vi "GetDefaultParams.vi"(8 "error in (no error)":errorcluster, 10 "Path":path, 11 "PmuTestFunctions.lvclass":refnum<class "PmuTestFunctions.lvclass">) -> (0 "error out":errorcluster, 3 "PmuTestFunctions.lvclass":refnum<class "PmuTestFunctions.lvclass">)   [LabVIEW 2014, in "Functions.lvlib" / "PmuTestFunctions.lvclass"]
uses:
  PmuTestFunctions.lvclass
  Typedefs/PmuTestParams.ctl
  FunctionBaseClass/FunctionBase.lvclass/FunctionBase.ctl
  PmuTestFunctions.lvclass/PmuTestFunctions.ctl
  FunctionBaseClass/Accessors/Read FunctionIniFilePath.vi
  Accessors/Write PmuTestParams.vi
  Accessors/Write T0.vi
  ArbitraryFunction/ArbitraryFunction.lvclass
  <vilib>/Utility/config.llb/NI_LVConfig.lvlib
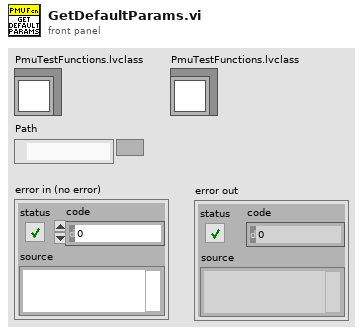
[diagram p1: front panel]
types:
  T1 = typedef "Functions.lvlib/PmuTestFunctions.lvclass/PmuTestParams.ctl" = dbl[][]
  T2 = typedef "NI_LVConfig.lvlib/Config Data RefNum.ctl" = refnum<k1>
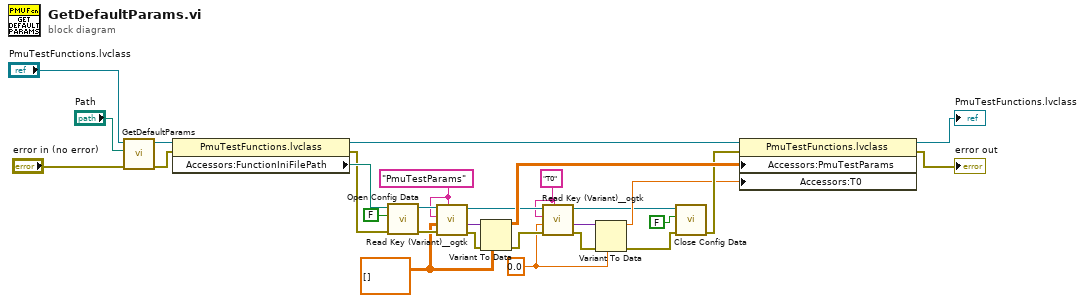
[diagram p0: block diagram]
diagram:
  w4 = 0.0
  w7 = "T0" ("section")
  w14 = T1 [] ("PmuTestParams")
  w17 = "PmuTestParams" ("section")
  n1 = call-parent "GetDefaultParams.vi"("error in (no error)"="error in (no error)", "Path"="Path", "ArbitraryFunction.lvclass"="PmuTestFunctions.lvclass") -> ("error out"=w24:errorcluster, "ArbitraryFunction.lvclass"=w29:refnum<class "PmuTestFunctions.lvclass">)  [unwired: 7 in]
  n2 = property class="PmuTestFunctions.lvclass"(reference=w29, error in=w24) -> (reference out=w25:refnum<class "PmuTestFunctions.lvclass">, error out=w20:errorcluster, "Accessors:FunctionIniFilePath"=w22:path)
  n3 = call <vilib>:"Open Config Data.vi"("error in (no error)"=w20, "create file if necessary (T)"=FALSE, "configuration file path"=w22) -> ("error out"=w19:errorcluster, "refnum"=w18:T2)  [unwired: 6 in, 1 out]
  n4 = call <userlib>:"Read Key (Variant)__ogtk.vi"("section"=w17, "error in (no error)"=w19, "type"=w14, "key (optional)"=w17, "refnum"=w18) -> ("error out"=w15:errorcluster, "key-value"=w16:variant, "refnum out"=w9:T2)  [unwired: 3 in, 1 out]
  n5 = Variant To Data(error in=w15, type=w14, Variant=w16) -> (data=w12:T1, error out=w8:errorcluster)
  n6 = call <userlib>:"Read Key (Variant)__ogtk.vi"("section"=w7, "error in (no error)"=w8, "type"=w4, "key (optional)"=w7, "refnum"=w9) -> ("error out"=w6:errorcluster, "key-value"=w5:variant, "refnum out"=w2:T2)  [unwired: 3 in, 1 out]
  n7 = Variant To Data(error in=w6, type=w4, Variant=w5) -> (data=w3:dbl, error out=w1:errorcluster)
  n8 = call <vilib>:"Close Config Data.vi"("error in (no error)"=w1, "write file if changed (T)"=FALSE, "refnum"=w2) -> ("error out"=w11:errorcluster)  [unwired: 7 in, 1 out]
  n9 = property class="PmuTestFunctions.lvclass"(reference=w25, error in=w11, "Accessors:PmuTestParams"=w12, "Accessors:T0"=w3) -> (reference out=→"PmuTestFunctions.lvclass":refnum<class "PmuTestFunctions.lvclass">, error out=→"error out":errorcluster)
